vi "Configure Band Selector Visibility.vi"(8 "error in (no error)":errorcluster, 10 "Number of Bands in":u8=4 min=3 max=6 step=1, 11 "Enum Refnum":refnum<vi>[](array[refnum])) -> (0 "error out":errorcluster, 2 "Number of Bands out":u8=4 min=3 max=6 step=1)   [LabVIEW 2018]
doc: "Configures the visibility of the resistor band selector controls on the Front Panel according to the selected number of bands.\n\nThe VI receives the <b>Number of Bands</b> and an array of <b>Enum Refnums</b>. It determines which band selectors must be visible for 3-, 4-, 5-, and 6-band resistor configurations and updates the <b>Visible</b> property of each Enum control.\n\nThe VI only configures Front Panel visibility. It does not modify the value or configuration of any band selector."
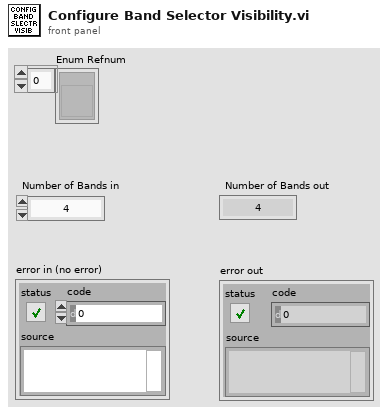
[diagram p1: front panel]
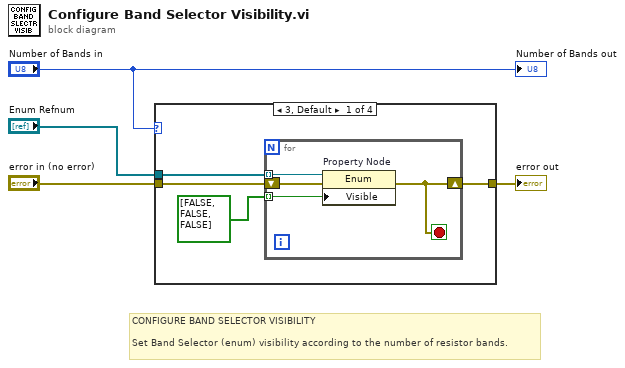
[diagram p0: block diagram]
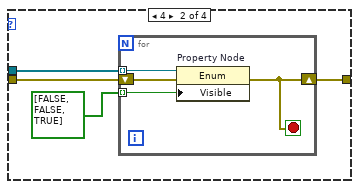
[diagram p2: hidden frame]
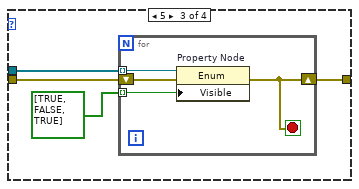
[diagram p3: hidden frame]
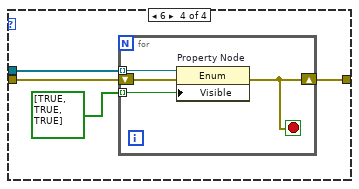
[diagram p4: hidden frame]
diagram:
  # "CONFIGURE BAND SELECTOR VISIBILITY\n\nSet Band Selector (enum) visibility according to the number of resistor bands."
  n1 = case shown="3, Default" "Number of Bands in" {
    tunnel: [w8 w14 w24 w31] -> w4
    tunnel: "error in (no error)" -> [w7 w15 w23 w32]
    tunnel: "Enum Refnum" -> [w6 w13 w22 w30]
    frame 3, Default {
      n2 = for {
        tunnel: bool[] [FALSE, FALSE, FALSE] -> [w9] mode=indexing
        shift-right: [w11] -> w8
        shift-left: w7 -> [w12]
        tunnel: w6 -> [w10] mode=indexing
        stop <- w11 stop-if-true
        n3 = property on="Property Node" class="Enum"(reference=w10, error in=w12, "Visible"=w9) -> (error out=w11:errorcluster)  [unwired: 1 out]
      }
    }
    frame 4 {
      n4 = for {
        tunnel: bool[] [FALSE, FALSE, TRUE] -> [w17] mode=indexing
        shift-right: [w19] -> w14
        shift-left: w15 -> [w20]
        tunnel: w13 -> [w18] mode=indexing
        stop <- w19 stop-if-true
        n5 = property on="Property Node" class="Enum"(reference=w18, error in=w20, "Visible"=w17) -> (error out=w19:errorcluster)  [unwired: 1 out]
      }
    }
    frame 5 {
      n6 = for {
        tunnel: bool[] [TRUE, FALSE, TRUE] -> [w25] mode=indexing
        shift-right: [w27] -> w24
        shift-left: w23 -> [w28]
        tunnel: w22 -> [w26] mode=indexing
        stop <- w27 stop-if-true
        n7 = property on="Property Node" class="Enum"(reference=w26, error in=w28, "Visible"=w25) -> (error out=w27:errorcluster)  [unwired: 1 out]
      }
    }
    frame 6 {
      n8 = for {
        tunnel: bool[] [TRUE, TRUE, TRUE] -> [w33] mode=indexing
        shift-right: [w35] -> w31
        shift-left: w32 -> [w36]
        tunnel: w30 -> [w34] mode=indexing
        stop <- w35 stop-if-true
        n9 = property on="Property Node" class="Enum"(reference=w34, error in=w36, "Visible"=w33) -> (error out=w35:errorcluster)  [unwired: 1 out]
      }
    }
  }
  "error out" <- w4
  "Number of Bands out" <- "Number of Bands in"
